vi "FdxCmdRxUDPChgDestPortCvi.vi"(8 "error in":errorcluster, 9 "RxUDPChgDestPort":cluster{"UdpHandle":u32, "UdpDst":u32}, 11 "InstrumentHandle_port":u32) -> (0 "error out":errorcluster, 3 "InstrumentHandle_port":u32)   [LabVIEW 2020, in "AIM664LV.lvlib"]
doc: "This function changes the UDP destination of a UDP queuing port. It can be used when\nreceiver is running"
uses:
  AIM664LV.lvlib
  AFDX_LibraryAdmin/FdxGlobalDllPath.vi
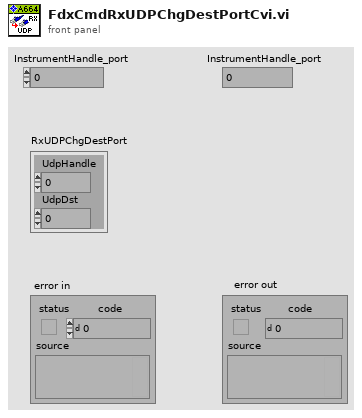
[diagram p1: front panel]
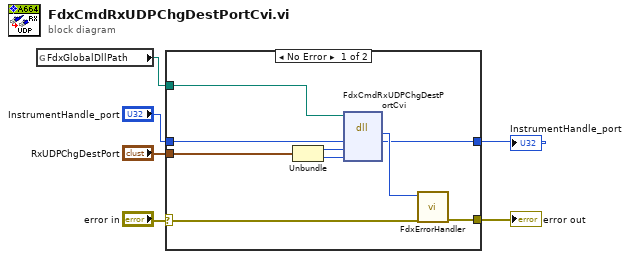
[diagram p0: block diagram]
diagram:
  n1 = global read "FdxGlobalDllPath.vi" "FdxGlobalDllPath"() -> (w4:path)
  n2 = case shown="No Error" "error in" {
    selector: "error in" -> [w14 w17]
    tunnel: [w15 w17] -> w6
    tunnel: w4 -> [w10 _]
    tunnel: "InstrumentHandle_port" -> [w9 w16]
    tunnel: [w8 w16] -> w2
    tunnel: "RxUDPChgDestPort" -> [w7 _]
    frame No Error {
      n3 = Unbundle(w7) -> ("UdpHandle"=w12:u32, "UdpDst"=w11:u32)
      n4 = dll-call lib="aim_fdx.19.dll" fn="FdxCmdRxUDPChgDestPortCvi"(path in=w10, "InstrumentHandle"=w9, "UdpHandle"=w12, "UdpDst"=w11) -> ("status"=w13:i32, "InstrumentHandle"=w8:u32)  [unwired: 4 in, 2 out]
      n5 = call "FdxErrorHandler.vi"("error in"=w14, "AIM Error"=w13) -> ("error out"=w15:errorcluster)  [unwired: 9 in]
    }
    frame Error {
    }
  }
  "error out" <- w6
  "InstrumentHandle_port" <- w2
